vi "Buttons_test.vi"() -> (2 "OUT":dbl)   [LabVIEW 2020]
uses:
  <vilib>/Rock Robotics/WPI/ThirdParty/Phoenix-LabVIEW/Motor Controller/Controls/CTRE_Phoenix_MotorControl_ControlMode.ctl
  GlobalVariables.vi
panel:
  out "Buttons 5":bool
  out "Buttons 4":bool
  out "Multiplicação":dbl
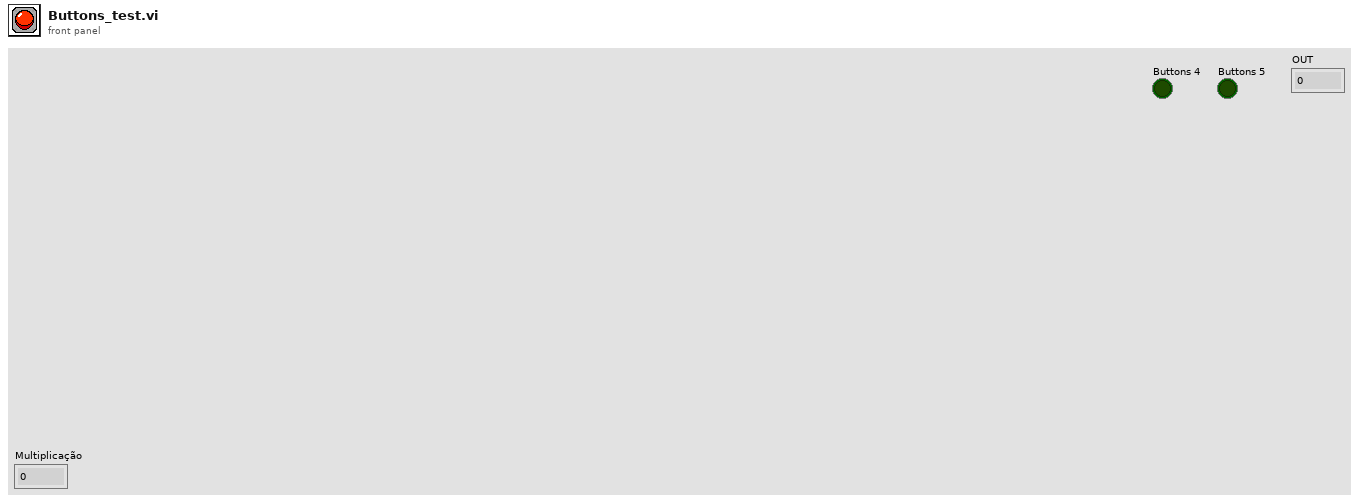
[diagram p1: front panel]
types:
  T1 = cluster{"Buttons[0]":bool, "Buttons[1]":bool, "Buttons[2]":bool, "Buttons[3]":bool, "Buttons[4]":bool, "Buttons[5]":bool, "Buttons[6]":bool, "Buttons[7]":bool, "Buttons[8]":bool}
  T2 = typedef "CTRE_Phoenix_MotorControl_ControlMode.ctl" = u16
  T3 = typedef "WPI_MotorControlDeviceRef.ctl" = cluster{"DeviceStatus":errorcluster, "Type":T4, "PWM":cluster{"PWM Channel":T5, "DeadBand":T6}, "CAN":cluster{"Device Number":u8, "SetOutput VI Ref":variant, "GetOutput VI Ref":variant, "Enable VI Ref":variant, "Disable VI Ref":variant, "Data":variant}, "Invert":bool, "DIO PWM":cluster{"PWM \"Enable\" Channel":T5, "DIOChannel":T7, "PWM Rate":dbl}}
  T4 = typedef "WPI_MotorControlType.ctl" = enum16{"PWM", "CAN", "DIO PWM"}
  T5 = typedef "FPGA_DIOPWMChannel.ctl" = enum8{"PWM 0", "PWM 1", "PWM 2", "PWM 3", "PWM 4", "PWM 5", "PWM 6", "PWM 7", "PWM 8", "PWM 9", "PWM MXP 0", "PWM MXP 1", "PWM MXP 2", "PWM MXP 3", "PWM MXP 4", "PWM MXP 5", "PWM MXP 6", "PWM MXP 7", "PWM MXP 8", "PWM MXP 9", "Invalid"}
  T6 = typedef "WPI_PWMDeadband.ctl" = cluster{"Name":string, "maxPositivePwm":i32, "minPositivePwm":i32, "centerPwm":i32, "maxNegativePwm":i32, "minNegativePwm":i32, "angularRange":u16}
  T7 = typedef "FPGA_DIOChannel.ctl" = enum8{"DIO 0", "DIO 1", "DIO 2", "DIO 3", "DIO 4", "DIO 5", "DIO 6", "DIO 7", "DIO 8", "DIO 9", "DIO MXP 0", "DIO MXP 1", "DIO MXP 2", "DIO MXP 3", "DIO MXP 4", "DIO MXP 5", "DIO MXP 6", "DIO MXP 7", "DIO MXP 8", "DIO MXP 9", "DIO MXP 10", "DIO MXP 11", "DIO MXP 12", "DIO MXP 13", "DIO MXP 14", "DIO MXP 15", "SPI Port CS1", "SPI Port CS2", "SPI Port CS3", "SPI Port MISO", "SPI Port MOSI", "Invalid"}
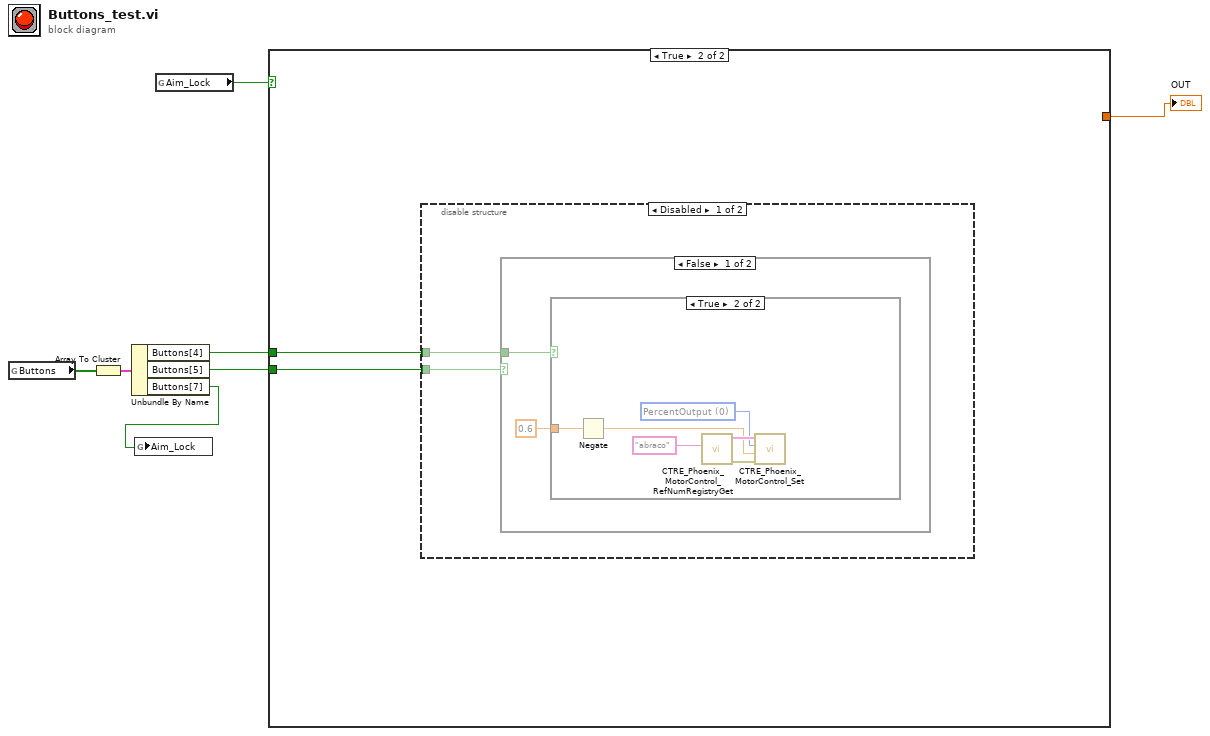
[diagram p0: block diagram]
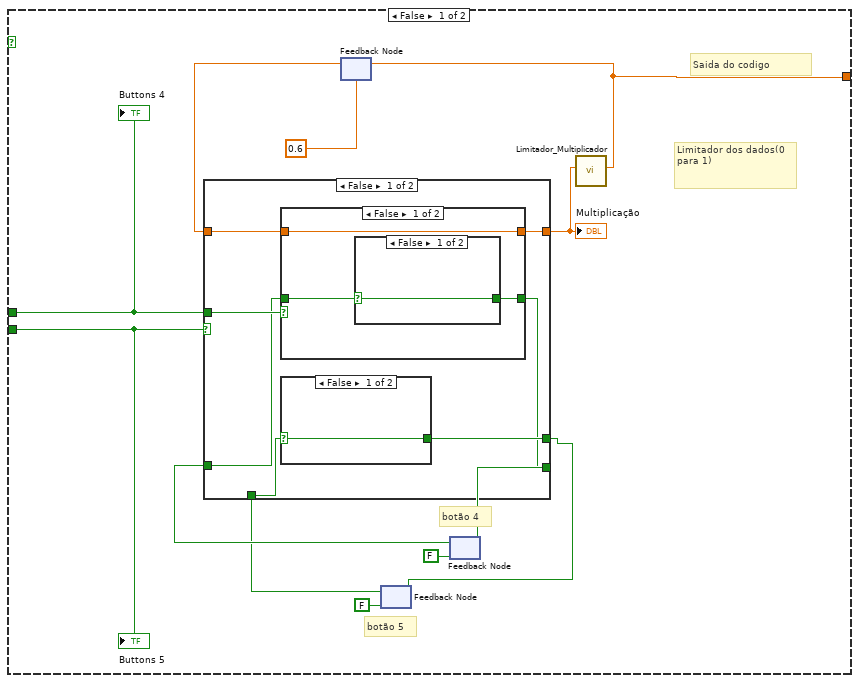
[diagram p2: hidden frame]
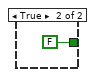
[diagram p3: hidden frame]
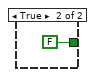
[diagram p4: hidden frame]
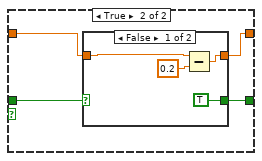
[diagram p5: hidden frame]
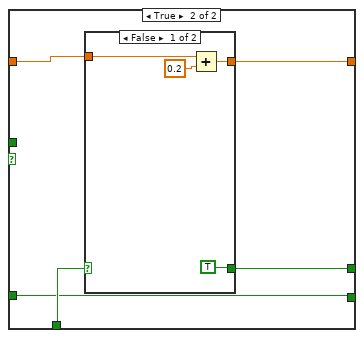
[diagram p7: hidden frame]
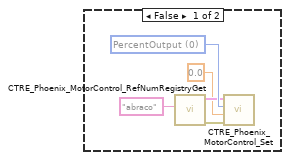
[diagram p9: hidden frame]
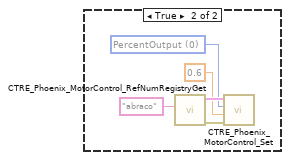
[diagram p10: hidden frame]
diagram:
  n1 = global read "GlobalVariables.vi" "Buttons"() -> (w4:bool[])
  n2 = Array To Cluster(array=w4) -> (cluster=w6:T1)
  n3 = Unbundle By Name(w6) -> ("Buttons[4]"=w2:bool, "Buttons[5]"=w3:bool, "Buttons[7]"=w5:bool)
  n4 = global write "GlobalVariables.vi" "Aim_Lock"(w5) -> ()
  n5 = global read "GlobalVariables.vi" "Aim_Lock"() -> (w7:bool)
  n6 = case shown="True" w7 {
    tunnel: w3 -> [w12 w55]
    tunnel: w2 -> [w11 w56]
    tunnel: [w8 _] -> w1
    frame False {
      # "Limitador dos dados(0 para 1)"
      # "Saida do codigo"
      # "botão 5"
      # "botão 4"
      n7 = feedback #1(0.6 ("y")) -> (w19:dbl)
      n8 = feedback #2(FALSE) -> (w16:bool)
      n9 = feedback #3(FALSE) -> (w17:bool)
      n10 = case shown="False" w12 {
        tunnel: w11 -> [w26 _]
        tunnel: [w24 w46] -> w18
        tunnel: w19 -> [w25 w47]
        tunnel: w16 -> [w23 w48]
        tunnel: [w22 w45] -> w10
        tunnel: w17 -> [w21 w44]
        tunnel: [w20 w44] -> w9
        frame False {
          n11 = case shown="False" w26 {
            tunnel: w25 -> [w31 w37]
            tunnel: [w31 w36] -> w24
            tunnel: w21 -> [w30 w35]
            tunnel: [w29 w34] -> w20
            frame False {
              n12 = case shown="False" w30 {
                selector: w30 -> [w32 _]
                tunnel: [w32 FALSE] -> w29
                frame False {
                }
                frame True {
                }
              }
            }
            frame True {
              n13 = case shown="False" w35 {
                selector: w35 -> [_ w42]
                tunnel: w37 -> [w40 w43]
                tunnel: [w39 w43] -> w36
                tunnel: [TRUE w42] -> w34
                frame False {
                  n14 = Subtract(x=w40, y=0.2) -> (x-y=w39:dbl)
                }
                frame True {
                }
              }
            }
          }
          n15 = case shown="False" w23 {
            selector: w23 -> [w27 _]
            tunnel: [w27 FALSE] -> w22
            frame False {
            }
            frame True {
            }
          }
        }
        frame True {
          n16 = case shown="False" w48 {
            selector: w48 -> [_ w53]
            tunnel: w47 -> [w51 w54]
            tunnel: [w50 w54] -> w46
            tunnel: [TRUE w53] -> w45
            frame False {
              n17 = Add(x=w51, y=0.2) -> (x+y=w50:dbl)
            }
            frame True {
            }
          }
        }
      }
      "Multiplicação" <- w18
      n18 = feedback-in #2(w10) -> ()
      n19 = feedback-in #3(w9) -> ()
      n20 = call "Limitador_Multiplicador.vi"("IN"=w18) -> ("OUT"=w8:dbl)  [unwired: 10 in]
      n21 = feedback-in #1(w8) -> ()
      "Buttons 4" <- w11
      "Buttons 5" <- w12
    }
    frame True {
      n22 = disable-structure shown="Disabled" {
        disable-tunnel: w56 -> [w58 _]
        disable-tunnel: w55 -> [w57 _]
        frame Disabled {
          n23 = case shown="False" w57 {
            tunnel: w58 -> [w59 _]
            frame False {
              n24 = case shown="True" w59 {
                tunnel: 0.6 ("Output") -> [_ w71]
                frame False {
                  w64 = T2 0 items=["PercentOutput"=0, "Position"=1, "Velocity"=2, "Current"=3, "Follower"=5, "MotionProfile"=6, "MotionMagic"=7, "MotionProfileArc"=10, "Disabled"=15] ("Control Mode")
                  n25 = call <vilib>:"CTRE_Phoenix_MotorControl_RefNumRegistryGet.vi"("refnum name"="abraco") -> ("error out"=w62:errorcluster, "PhoenixMotorControlDevRef"=w63:T3)  [unwired: 9 in]
                  n26 = call <vilib>:"CTRE_Phoenix_MotorControl_Set.vi"("error in (no error)"=w62, "Output"=0.0, "Control Mode"=w64, "PhoenixMotorControlDevRef"=w63) -> ()  [unwired: 6 in, 2 out]
                }
                frame True {
                  w67 = T2 0 items=["PercentOutput"=0, "Position"=1, "Velocity"=2, "Current"=3, "Follower"=5, "MotionProfile"=6, "MotionMagic"=7, "MotionProfileArc"=10, "Disabled"=15] ("Control Mode")
                  n27 = Negate(x=w71) -> (-x=w66:dbl)
                  n28 = call <vilib>:"CTRE_Phoenix_MotorControl_RefNumRegistryGet.vi"("refnum name"="abraco") -> ("error out"=w69:errorcluster, "PhoenixMotorControlDevRef"=w68:T3)  [unwired: 9 in]
                  n29 = call <vilib>:"CTRE_Phoenix_MotorControl_Set.vi"("error in (no error)"=w69, "Output"=w66, "Control Mode"=w67, "PhoenixMotorControlDevRef"=w68) -> ()  [unwired: 6 in, 2 out]
                }
              }
            }
            frame True {
              w73 = T2 0 items=["PercentOutput"=0, "Position"=1, "Velocity"=2, "Current"=3, "Follower"=5, "MotionProfile"=6, "MotionMagic"=7, "MotionProfileArc"=10, "Disabled"=15] ("Control Mode")
              n30 = call <vilib>:"CTRE_Phoenix_MotorControl_RefNumRegistryGet.vi"("refnum name"="abraco") -> ("error out"=w75:errorcluster, "PhoenixMotorControlDevRef"=w76:T3)  [unwired: 9 in]
              n31 = call <vilib>:"CTRE_Phoenix_MotorControl_Set.vi"("error in (no error)"=w75, "Output"=0.6, "Control Mode"=w73, "PhoenixMotorControlDevRef"=w76) -> ()  [unwired: 6 in, 2 out]
            }
          }
        }
        frame Enabled {
        }
      }
    }
  }
  "OUT" <- w1
